vi "Create Property List.vi"(8 "error in":errorcluster, 11 "Property Nodes In":refnum<k20>) -> (0 "error out":errorcluster, 2 "Properties out":refnum<class "Property.lvclass">[](array[class]), 3 "Property Nodes out":refnum<k20>)   [LabVIEW 2024, in "Parser.lvlib" / "Property.lvclass"]
uses:
  Property.lvclass
  <vilib>/xml/Close Reference(Node).vi
  Parser.lvlib
  <vilib>/xml/NI_XML.lvlib
  <resource>/objmgr/DOMUserDefRef.rc
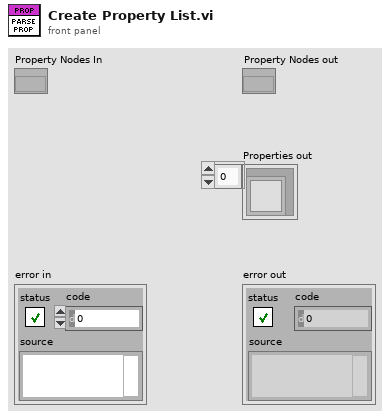
[diagram p1: front panel]
types:
  T1 = typedef "Parser.lvlib/Property.lvclass/Property Type.ctl" = enum16{"Boolean", "Double", "String", "Path", "Dictionary", "DependentFile", "I16", "I32", "I64", "U16", "U32", "U64", "BooleanArray", "DoubleArray", "StringArray", "I16Array", "I32Array", "I64Array", "U16Array", "U32Array", "U64Array", "Variant"}
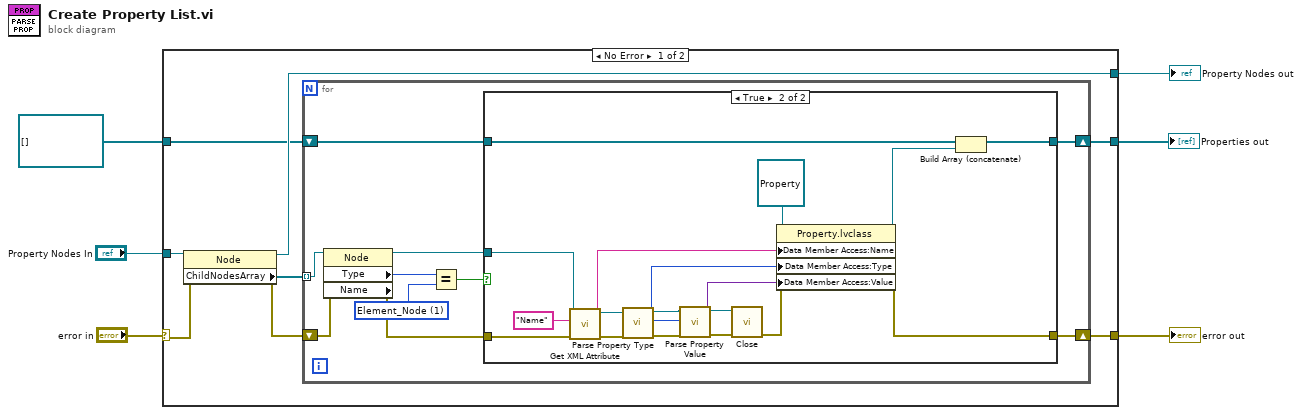
[diagram p0: block diagram]
diagram:
  n1 = case shown="No Error" "error in" {
    selector: "error in" -> [w13 w47]
    tunnel: [w14 w47] -> w5
    tunnel: "Property Nodes In" -> [w11 w46]
    tunnel: [w9 w46] -> w3
    tunnel: refnum<class "Property.lvclass">[] [] ("reference out 2") -> [w8 w45]
    tunnel: [w7 w45] -> w1
    frame No Error {
      n2 = property class="Node"(reference=w11, error in=w13) -> (reference out=w9:refnum<k20>, error out=w12:errorcluster, "ChildNodesArray"=w10:refnum<k20>[])
      n3 = for {
        shift-right: [w24] -> w14
        shift-left: w12 -> [w23]
        tunnel: w10 -> [w21] mode=indexing
        shift-right: [w16] -> w7
        shift-left: w8 -> [w17]
        w18 = 1 items=["Element_Node"=1, "Attribute_Node"=2, "Text_Node"=3, "CDATASection_Node"=4, "EntityReference_Node"=5, "Entity_Node"=6, "ProcessingInstruction_Node"=7, "Comment_Node"=8, "Document_Node"=9, "DocumentType_Node"=10, "DocumentFragment_Node"=11, "Notation_Node"=12] ("Node Type")
        n4 = property class="Node" props=["Type", "Name"](reference=w21, error in=w23) -> (reference out=w15:refnum<k20>, error out=w22:errorcluster, "Type"=w19:i32)  [unwired: 1 out]
        n5 = Equal?(x=w19, y=w18) -> (x = y?=w20:bool)
        n6 = case shown="True" w20 {
          tunnel: [w26 w40] -> w24
          tunnel: w22 -> [w26 w39]
          tunnel: w17 -> [w25 w30]
          tunnel: [w25 w29] -> w16
          tunnel: w15 -> [_ w27]
          frame False {
          }
          frame True {
            n7 = call "Get XML Attribute.vi"("error in"=w39, "Attribute Name"="Name", "XML Node"=w27) -> ("error out"=w44:errorcluster, "Attribute Value"=w34:string, "XML Node out"=w37:refnum<k20>)  [unwired: 6 in]
            n8 = call "Parse Property Type.vi"("error in"=w44, "Node in"=w37) -> ("error out"=w43:errorcluster, "Property Type"=w33:T1, "Child Node out"=w36:refnum<k20>)  [unwired: 7 in]
            n9 = call "Parse Property Value.vi"("error in"=w43, "Property Type"=w33, "Node in"=w36) -> ("error out"=w42:errorcluster, "Property Value"=w32:variant, "Node out"=w31:refnum<k20>)  [unwired: 6 in]
            n10 = call-poly <vilib>:"Close.vi"("error in (no error)"=w42, "node"=w31) -> ("error out"=w41:errorcluster)  [unwired: 7 in]
            n11 = property class="Property.lvclass"(reference=refnum<class "Property.lvclass"> refnum ("Parser.lvlib:Property.lvclass"), error in=w41, "Data Member Access:Name"=w34, "Data Member Access:Type"=w33, "Data Member Access:Value"=w32) -> (reference out=w28:refnum<class "Property.lvclass">, error out=w40:errorcluster)
            n12 = Build Array (concatenate)(w30, w28) -> (w29:refnum<class "Property.lvclass">[])
          }
        }
      }
    }
    frame Error {
    }
  }
  "error out" <- w5
  "Property Nodes out" <- w3
  "Properties out" <- w1
